vi "Get Morphology Structuring Element (Elipse).vi"(7 "Anchor (Default: -1, -1 Use Centre)":T1={"x"=-1, "y"=-1}, 8 "error in (no error)":errorcluster, 11 "Size":T2) -> (0 "error out":errorcluster, 3 "Structuring Element":bool[][](array[boolean]))   [LabVIEW 2020, in "image.lvlib"]
doc: "Create a Structuring Element for use with the Image Morphology operations."
uses:
  image.lvlib
  common/Image Size (Integer).ctl
  common/Image Point (Integer).ctl
  MorphologyStructuredElementShape.ctl
  <vilib>/Utility/error.llb/Error Cluster From Error Code.vi
  common/common.lvlib
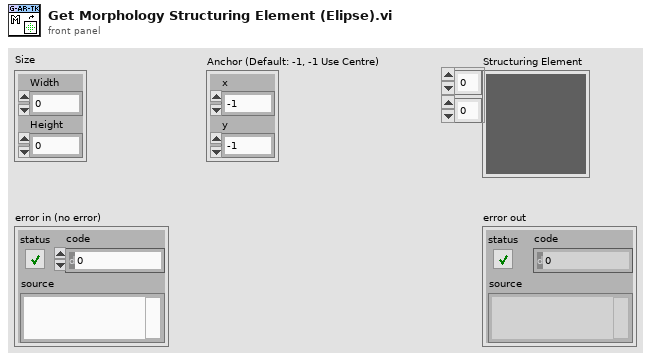
[diagram p1: front panel]
types:
  T1 = typedef "common.lvlib/Image Point (Integer).ctl" = cluster{"x":i32, "y":i32}
  T2 = typedef "common.lvlib/Image Size (Integer).ctl" = cluster{"Width":u16, "Height":u16}
  T3 = typedef "image.lvlib/MorphologyStructuredElementShape.ctl" = enum16{"Rect", "Cross", "Elipse"}
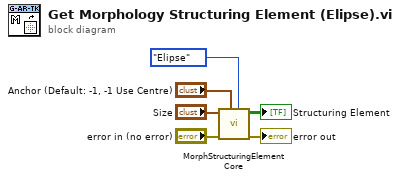
[diagram p0: block diagram]
diagram:
  n1 = call "MorphStructuringElementCore.vi"("Shape"=MorphologyStructuredElementShape."Elipse", "Anchor (Default: -1, -1 Use Centre)"="Anchor (Default: -1, -1 Use Centre)", "error in (no error)"="error in (no error)", "Size"="Size") -> ("error out"=→"error out":errorcluster, "Structuring Element"=→"Structuring Element":bool[][])  [unwired: 6 in]
